vi "TestConfig.vi"() -> ()   [LabVIEW 2014]
uses:
  Config.lvclass
panel:
  out "ErrorArray":errorcluster[](array[cluster])
  in  "btnSettings":bool
  in  "btnStop":bool
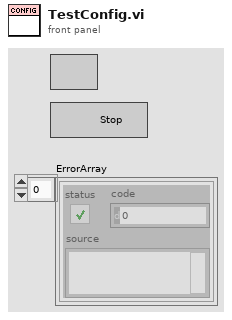
[diagram p1: front panel]
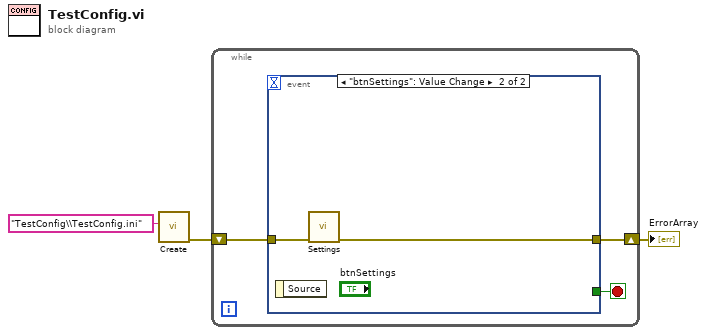
[diagram p0: block diagram]
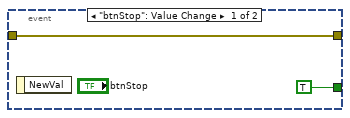
[diagram p2: hidden frame]
diagram:
  n1 = call "Create.vi"("name or relative path"="TestConfig\\TestConfig.ini") -> ("ErrorArray"=w2:errorcluster[])  [unwired: 9 in, 1 out]
  n2 = while {
    shift-right: [w5] -> w1
    shift-left: w2 -> [w6]
    stop <- w4 stop-if-true
    n3 = event shown="[1] \"btnSettings\": Value Change" {
      selector: _ -> [_ _]
      dyn-events: _ -> [_ _]
      timeout: _ -> [_ _]
      tunnel: [w8 w9] -> w5
      tunnel: w6 -> [w8 w10]
      tunnel: [TRUE _] -> w4
      event "btnStop": Value Change {
        n4 = event-data() -> ()  [unwired: 1 in, 1 out]
      }
      event "btnSettings": Value Change {
        n5 = event-data() -> ()  [unwired: 1 in, 1 out]
        n6 = call "Settings.vi"("ErrorArray"=w10) -> ("ErrorArray"=w9:errorcluster[])  [unwired: 10 in]
      }
    }
  }
  "ErrorArray" <- w1
